vi "LINX - SSD1306 OLED.vi"() -> ()   [LabVIEW 2020]
doc: "This example demonstrates how to control an OLED using the SSD1306 OLED driver."
uses:
  vi.lib/MakerHub/LINX/Public/Sensors/Display/SSD1306/Private/SSD1306 Config.ctl
  vi.lib/MakerHub/LINX/Public/Utilities/Open Serial.vi
  vi.lib/MakerHub/LINX/LMH-LINX.lvlib
  vi.lib/MakerHub/LINX/Public/Sensors/Display/SSD1306/SSD1306.lvlib
panel:
  out "Image":picture
  in  "Image Path (128x32 PNG)":path
  in  "Stop Button":bool
  in  "SSD1306 Channels":T1={"SPI Channel (0)"=0, "VDD Channel"=38, "VBAT Channel"=40, "RESET Channel"=10, "DC Channel"=39, "SPI CS (3)"=0}
  in  "Serial Port":refnum<visa-resource-name>="COM3"
  # "SSD1306 Example\n\nThis example demonstrates how draw a 128 x 32 pixel PNG on an OLED driven by the SSD1306.\n\nNote: This example is configured to use a serial interface but can easily be modified\nto use TCP or run on myRIO.\n\nInstructions\n1. Select the COM Port associated with the LINX Device.\n2. Configure the SPI and DIO channels corresponding to the SSD1306.\n3. Click the Run Arrow.\n4. Click the browse button the Image Path control and select a 128 x 32 PNG file.\n5. Notice the display updates with the selected image."
  # "Configuration"
  # "Image"
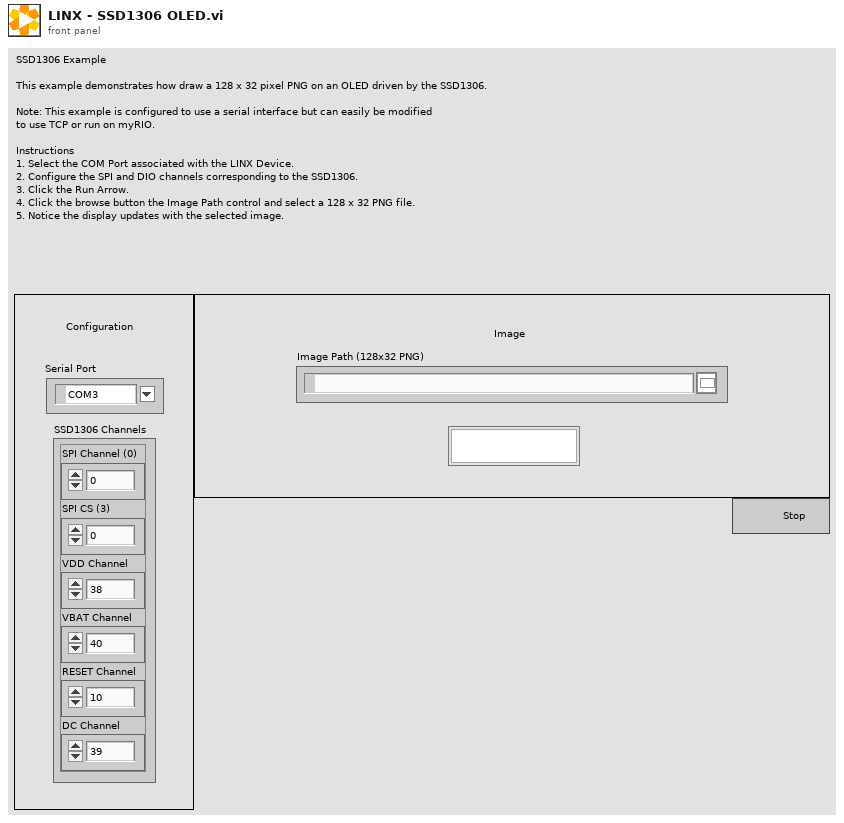
[diagram p1: front panel]
types:
  T1 = typedef "LMH-LINX.lvlib/SSD1306.lvlib/SSD1306 Config.ctl" = cluster{"SPI Channel (0)":u8, "VDD Channel":u8, "VBAT Channel":u8, "RESET Channel":u8, "DC Channel":u8, "SPI CS (3)":u8}
  T2 = typedef "LMH-LINX.lvlib/LINX Ref.ctl" = cluster{"IO":T3, "Interface":T4, "LINX Device Config":T5}
  T3 = typedef "LMH-LINX.lvlib/Platform.ctl" = enum16{"Remote", "Local"}
  T4 = typedef "LMH-LINX.lvlib/Interface.ctl" = enum16{"Serial", "TCP"}
  T5 = typedef "Device.lvlib/LINX Device Config.ctl" = cluster{"Interface":T4, "COM Port":refnum<visa-resource-name>, "TCP Configuration":T6, "Device Family":u8, "Device ID":u8, "Device Name":string, "TCP Ref":refnum<k5>, "Channels":T7}
  T6 = typedef "Device.lvlib/TCP Config.ctl" = cluster{"IP Address":string, "Port":u16}
  T7 = typedef "LMH-LINX.lvlib/Channels.ctl" = cluster{"DI":u8[], "DO":u8[], "AI":u8[], "AO":u8[], "PWM":u8[], "QE":u8[], "UART":u8[], "I2C 2":u8[], "SPI":u8[], "CAN":u8[], "Servo":u8[], "AI Ref (V)":dbl, "AI Resolution (Bits)":u8, "AO Ref (V)":dbl, "AO Resolution (Bits)":u8}
  T8 = typedef "imagedata.ctl" = cluster{"image type":i32, "image depth":i32, "image":u8[], "mask":u8[], "colors":u32[], "Rectangle":cluster{"left":i16, "top":i16, "right":i16, "bottom":i16}}
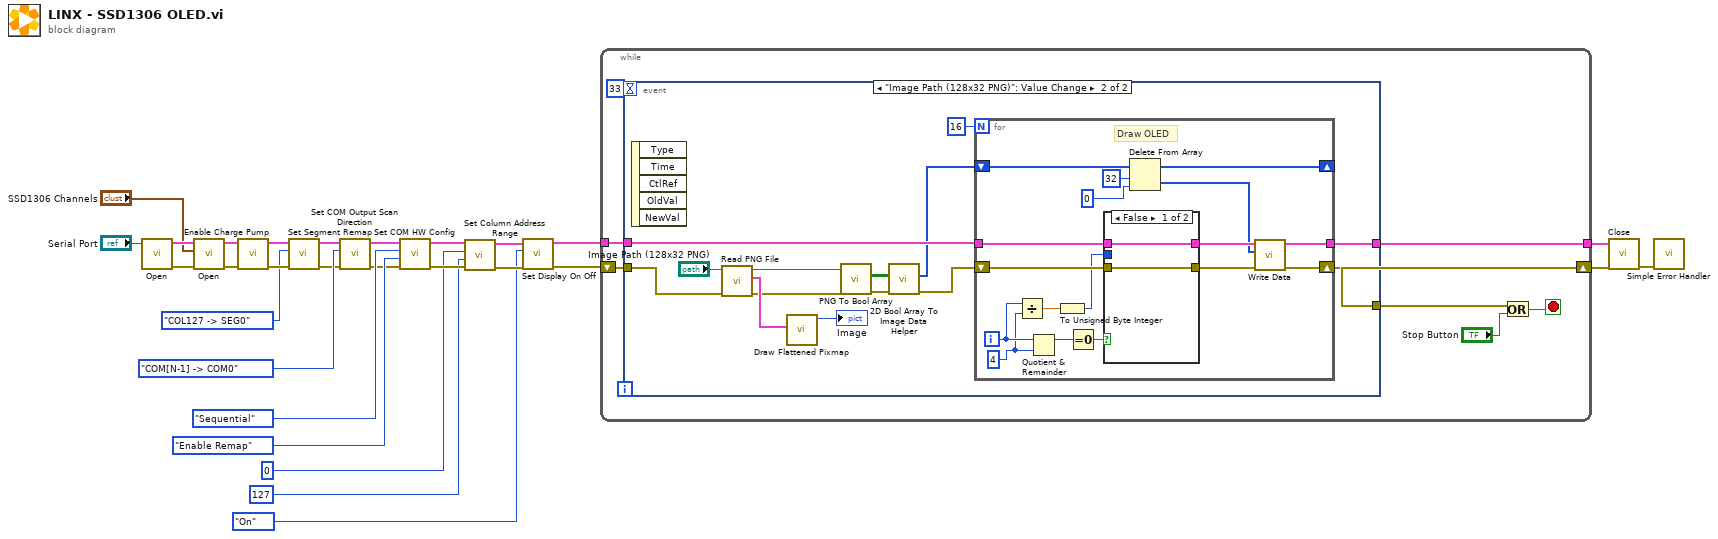
[diagram p0: block diagram]
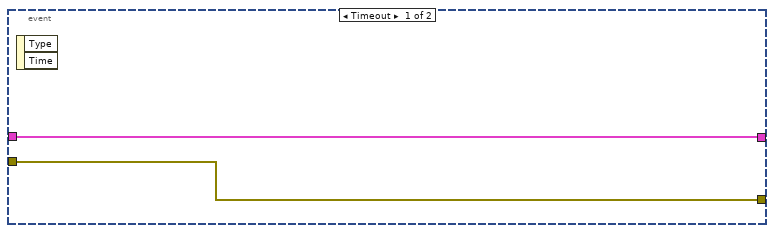
[diagram p2: hidden frame]
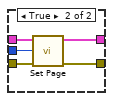
[diagram p3: hidden frame]
diagram:
  n1 = call-poly "Open.vi"("Serial Port"="Serial Port") -> ("Error Out"=w25:errorcluster, "LINX Resource"=w26:T2)  [unwired: 8 in, 1 out]
  n2 = call "Open.vi"("Error In"=w25, "SSD1306 Channels"="SSD1306 Channels", "LINX Resource"=w26) -> ("Error Out"=w22:errorcluster, "LINX Resource"=w23:T2)  [unwired: 7 in]
  n3 = call "Enable Charge Pump.vi"("Error In"=w22, "LINX Resource"=w23) -> ("Error Out"=w21:errorcluster, "LINX Resource"=w20:T2)  [unwired: 8 in]
  n4 = call "Set Segment Remap.vi"("Error In"=w21, "Segment Remap"=enum8{"COL 0 -> SEG0", "COL127 -> SEG0"}."COL127 -> SEG0", "LINX Resource"=w20) -> ("Error Out"=w14:errorcluster, "LINX Resource"=w15:T2)  [unwired: 7 in]
  n5 = call "Set COM Output Scan Direction.vi"("Error In"=w14, "COM Direction"=enum8{"COM0 -> COM[N-1]", "COM[N-1] -> COM0"}."COM[N-1] -> COM0", "LINX Resource"=w15) -> ("Error Out"=w12:errorcluster, "LINX Resource"=w13:T2)  [unwired: 7 in]
  n6 = call "Set COM HW Config.vi"("Error In"=w12, "COM Left/Right Remap"=enum8{"Disable Remap", "Enable Remap"}."Enable Remap", "COM Pin Config"=enum8{"Sequential", "Alternative"}."Sequential", "LINX Resource"=w13) -> ("Error Out"=w11:errorcluster, "LINX Resource"=w10:T2)  [unwired: 6 in]
  n7 = call "Set Column Address Range.vi"("Error In"=w11, "Column End Address"=u8 127 ("Column Start Address"), "Column Start Address"=u8 0, "LINX Resource"=w10) -> ("Error Out"=w7:errorcluster, "LINX Resource"=w6:T2)  [unwired: 6 in]
  n8 = call "Set Display On Off.vi"("Error In"=w7, "Display On/Off"=enum8{"Off", "On"}."On", "LINX Resource"=w6) -> ("Error Out"=w4:errorcluster, "LINX Resource"=w3:T2)  [unwired: 7 in]
  n9 = while {
    tunnel: w3 -> [w33]
    shift-right: [w32] -> w2
    shift-left: w4 -> [w30]
    tunnel: [w31] -> w1
    stop <- w35 stop-if-true
    n10 = event shown="[1] \"Image Path (128x32 PNG)\": Value Change" {
      selector: _ -> [_ _]
      dyn-events: _ -> [_ _]
      timeout: 33 -> [_ _]
      tunnel: w33 -> [w36 w50]
      tunnel: [w37 w49] -> w32
      tunnel: [w36 w48] -> w31
      tunnel: w30 -> [w37 w40]
      event Timeout {
        n11 = event-data() -> ()  [unwired: 1 in, 2 out]
      }
      event "Image Path (128x32 PNG)": Value Change {
        n12 = event-data() -> ()  [unwired: 1 in, 5 out]
        n13 = call <vilib>:"Read PNG File.vi"("error in (no error)"=w40, "path to PNG file"="Image Path (128x32 PNG)") -> ("error out"=w39:errorcluster, "image data"=w43:T8, "path"=w38:path)  [unwired: 7 in]
        n14 = call <vilib>:"Draw Flattened Pixmap.vi"("image data"=w43) -> ("new picture"=→"Image":picture)  [unwired: 8 in]
        n15 = call "PNG To Bool Array.vi"("Error In"=w39, "path to PNG file"=w38) -> ("Error Out"=w47:errorcluster, "Array"=w45:bool[][])  [unwired: 8 in]
        n16 = call "2D Bool Array To Image Data Helper.vi"("Error In"=w47, "Image Data"=w45) -> ("Error Out"=w46:errorcluster, "Image Data"=w44:u8[])  [unwired: 8 in]
        n17 = for {
          N: 16 -> [_]
          tunnel: w50 -> [w61]
          shift-right: [w57] -> _
          shift-left: w44 -> [w58]
          shift-right: [w53] -> w49
          shift-left: w46 -> [w66]
          tunnel: [w52] -> w48
          i -> [w65]
          w64 = 4 ("y")
          # "Draw OLED"
          n18 = Divide(x=w65, y=w64) -> (x/y=w63:dbl)
          n19 = Quotient & Remainder(x=w65, y=w64) -> (x-y*floor(x/y)=w68:i32)  [unwired: 1 out]
          n20 = To Unsigned Byte Integer(number=w63) -> (unsigned 8bit integer=w62:u8)
          n21 = Equal To 0?(x=w68) -> (x = 0?=w67:bool)
          n22 = case shown="False" w67 {
            tunnel: w66 -> [w69 w75]
            tunnel: w62 -> [_ w74]
            tunnel: w61 -> [w70 w73]
            tunnel: [w69 w72] -> w60
            tunnel: [w70 w71] -> w59
            frame False {
            }
            frame True {
              n23 = call "Set Page.vi"("Error In"=w75, "Page Address"=w74, "LINX Resource"=w73) -> ("Error Out"=w72:errorcluster, "LINX Resource"=w71:T2)  [unwired: 7 in]
            }
          }
          n24 = Delete From Array(array=w58, length=32, index=0) -> (deleted portion=w54:u8[], array with subset deleted=w57:u8[])
          n25 = call "Write Data.vi"("Error In"=w60, "Data"=w54, "LINX Resource"=w59) -> ("Error Out"=w53:errorcluster, "LINX Resource"=w52:T2)  [unwired: 7 in]
        }
      }
    }
    n26 = Or(x=w32, y="Stop Button") -> (x .or. y?=w35:bool)
  }
  n27 = call "Close.vi"("Error In"=w2, "LINX Resource"=w1) -> ("Error Out"=w27:errorcluster)  [unwired: 9 in]
  n28 = call <vilib>:"Simple Error Handler.vi"("error in (no error)"=w27) -> ()  [unwired: 4 in, 5 out]
